vi "Set Defaults from Strings.vi"(8 "error in (no error)":errorcluster, 10 "Default Strings":string[](array[string]), 11 "StringGroup in":refnum<class "StringGroup.lvclass">) -> (0 "error out":errorcluster, 3 "StringGroup out":refnum<class "StringGroup.lvclass">)   [LabVIEW 2020, in "Vecto.lvlib" / "StringGroup.lvclass"]
uses:
  StringGroup.lvclass
  StringGroup.lvclass/StringGroup.ctl
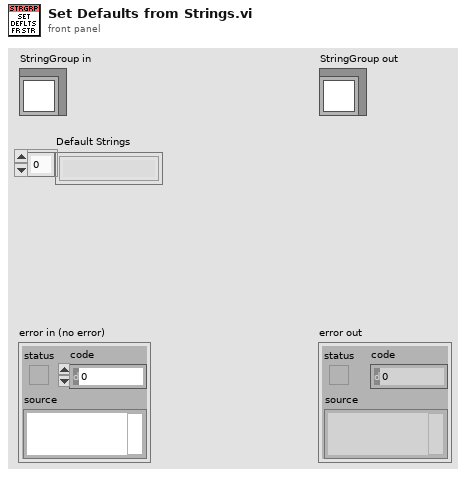
[diagram p1: front panel]
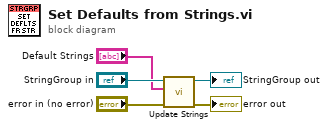
[diagram p0: block diagram]
diagram:
  n1 = call "Update Strings.vi"("error in (no error)"="error in (no error)", "Strings"="Default Strings", "StringGroup in"="StringGroup in") -> ("error out"=→"error out":errorcluster, "StringGroup out"=→"StringGroup out":refnum<class "StringGroup.lvclass">)  [unwired: 7 in]
